vi "Activate Gas Board.vi"(7 "CAN Interface":string="GAS", 8 "error in (no error)":errorcluster) -> (0 "error out":errorcluster, 3 "Session Handle out":T1 caption="Gas")   [LabVIEW 2015, in "Gas.lvclass"]
uses:
  Gas.lvclass
  Typedefs/Session Handle.ctl
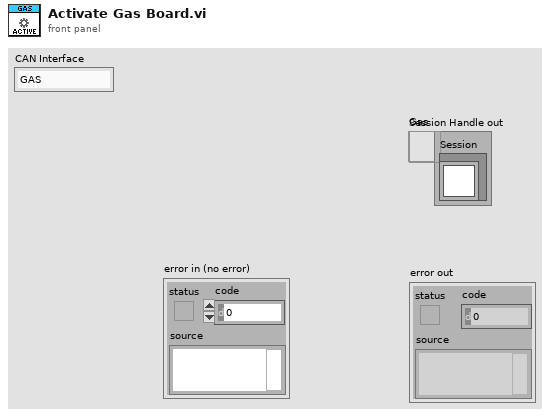
[diagram p1: front panel]
types:
  T1 = typedef "Gas.lvclass/Session Handle.ctl" = refnum<data-value>
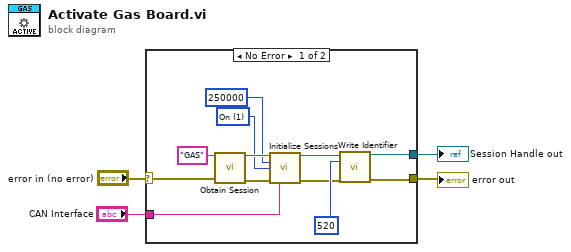
[diagram p0: block diagram]
diagram:
  n1 = case shown="No Error" "error in (no error)" {
    selector: "error in (no error)" -> [w10 w17]
    tunnel: [w7 w17] -> w4
    tunnel: [w6 _] -> w2
    tunnel: "CAN Interface" -> [w5 _]
    frame No Error {
      w13 = u32 1 items=["Off", "On"] ("Termination")
      n2 = call "Obtain Session.vi"("Session  Name ()"="GAS", "error in (no error)"=w10) -> ("Session Handle"=w15:T1, "error out"=w16:errorcluster)  [unwired: 12 in]
      n3 = call "Initialize Sessions.vi"("Session Handle in"=w15, "Baud Rate"=u32 250000, "Termination"=w13, "error in (no error)"=w16, "CAN Interface"=w5) -> ("Session Handle Out"=w8:T1, "error out"=w9:errorcluster)  [unwired: 9 in]
      n4 = call "Write Identifier.vi"("Session Handle in"=w8, "identifier"=u16 520, "error in (no error)"=w9) -> ("Session Handle out"=w6:T1, "error out"=w7:errorcluster)  [unwired: 11 in]
    }
    frame Error {
    }
  }
  "error out" <- w4
  "Session Handle out" <- w2
